vi "generate_gauss_curve.vi"(5 "num points":u32, 6 "offset":dbl, 7 "Spread":dbl, 8 "Center":dbl, 9 "Amplitude":dbl) -> (2 "Y Values":dbl[](array[numeric]), 3 "X Values":dbl[](array[numeric]))   [LabVIEW 2014]
doc: "Takes fit parameters (typically from gauss_fit.vi) and produces a gaussuan curve based on those coefficients."
panel:
  out "XY Graph":cluster{dbl[], dbl[]}(graph)
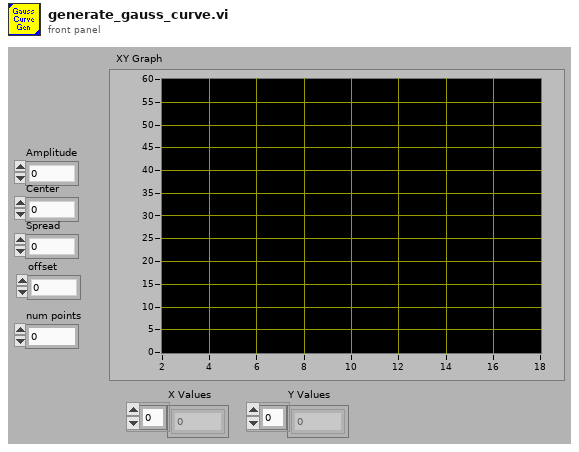
[diagram p1: front panel]
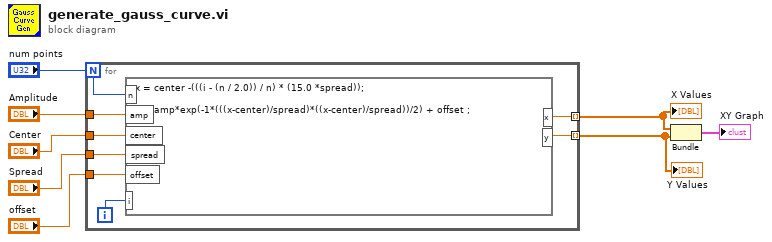
[diagram p0: block diagram]
diagram:
  n1 = for {
    N: "num points" -> [w11]
    tunnel: "Amplitude" -> [w16]
    tunnel: "Center" -> [w13]
    tunnel: "Spread" -> [w14]
    tunnel: [w15] -> w4 mode=indexing
    tunnel: "offset" -> [w12]
    tunnel: [w9] -> w2 mode=indexing
    i -> [w10]
    n2 = formula code="x = center -(((i - (n / 2.0)) / n) * (15.0 *spread));\n\ny = amp*exp(-1*(((x-center)/spread)*((x-center)/spread))/2) + offset ;"("amp"=w16, "center"=w13, "spread"=w14, "i"=w10, "offset"=w12, "n"=w11) -> ("y"=w15:dbl, "x"=w9:dbl)
  }
  "X Values" <- w2
  "Y Values" <- w4
  n3 = Bundle(w2, w4) -> (→"XY Graph":cluster{dbl[], dbl[]})  [unwired: 1 in]
